vi "Save.vi"(8 "error in (no error)":errorcluster, 11 "User Preferences File in":refnum<class "User Preferences File.lvclass">) -> (0 "error out":errorcluster, 3 "User Preferences File out":refnum<class "User Preferences File.lvclass">)   [LabVIEW 2020, in "RxnRover.lvlib" / "User Preferences File.lvclass"]
doc: "Format the User Preferences file as a readable JSON file and write it to disk."
uses:
  User Preferences File.lvclass
  User Preferences File.lvclass/User Preferences File.ctl
  File IO/JSON Utilities/JSON Utilities.lvlib
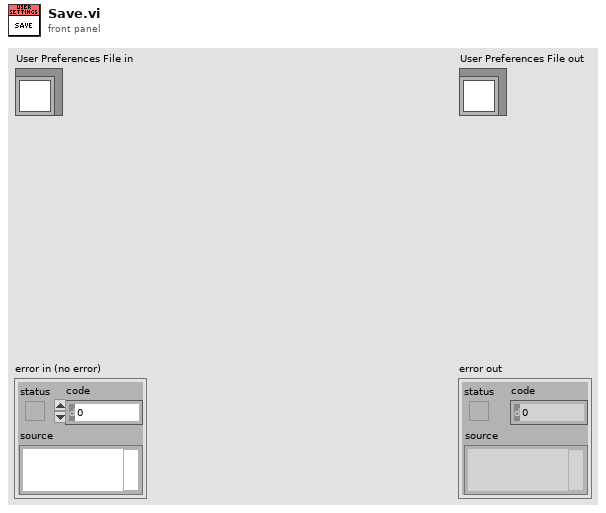
[diagram p1: front panel]
types:
  T1 = enum16{"open", "replace", "create", "open or create", "replace or create", "replace or create with confirmation"}
  T2 = typedef "RxnRover.lvlib/User Preferences File.lvclass/User Preferences Cluster.ctl" = cluster{"Max Recent Experiments":dbl, "Recent Experiments":string[]}
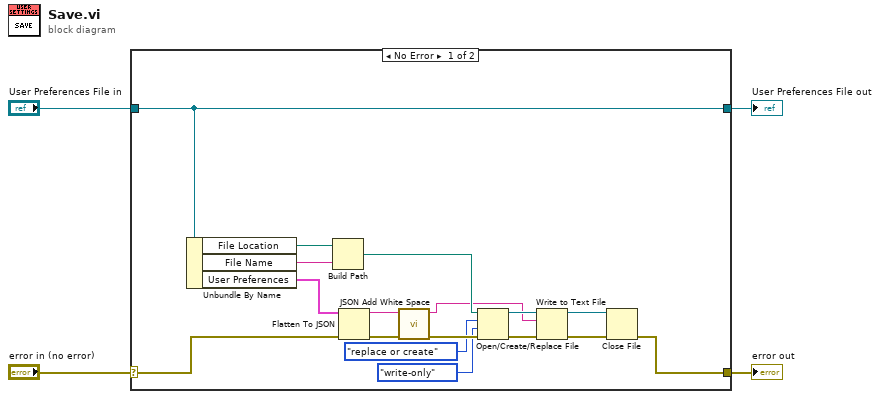
[diagram p0: block diagram]
diagram:
  n1 = case shown="No Error" "error in (no error)" {
    selector: "error in (no error)" -> [w19 w23]
    tunnel: [w11 w23] -> w3
    tunnel: [w21 w22] -> w1
    tunnel: "User Preferences File in" -> [w21 w22]
    frame No Error {
      n2 = Unbundle By Name(w21) -> ("File Location"=w14:path, "File Name"=w15:string, "User Preferences"=w20:T2)
      n3 = Build Path(base path=w14, name or relative path=w15) -> (appended path=w6:path)
      n4 = Flatten To JSON(anything=w20, error in (no error)=w19) -> (JSON string=w16:string, 11:w18:errorcluster)  [unwired: 1 in]
      n5 = call "JSON Add White Space.vi"("error in (no error)"=w18, "JSON string"=w16) -> ("error out"=w17:errorcluster, "Modified JSON string"=w5:string)  [unwired: 8 in]
      n6 = Open/Create/Replace File(file path (use dialog)=w6, error in=w17, operation (0:open)=T1."replace or create", access (0:read/write)=enum16{"read/write", "read-only", "write-only"}."write-only") -> (refnum out=w9:refnum<file>, error out=w12:errorcluster)  [unwired: 2 in, 1 out]
      n7 = Write to Text File(file (use dialog)=w9, text=w5, error in=w12) -> (refnum out=w10:refnum<file>, error out=w13:errorcluster)  [unwired: 1 in, 1 out]
      n8 = Close File(refnum=w10, error in=w13) -> (error out=w11:errorcluster)  [unwired: 1 out]
    }
    frame Error {
    }
  }
  "error out" <- w3
  "User Preferences File out" <- w1
